vi "G4BaseTemplate_Singleton_5x6x5_GetProperty.vi"(11 "Error In":errorcluster) -> (8 "Property":dbl, 15 "Error Out":errorcluster)   [LabVIEW 2020]
uses:
  <resource>/Framework/Providers/Open_GDS/ClassProviders/Provider_EndevoGOOP400/Templates/G4BaseTemplate_Singleton_5x6x5/G4BaseTemplate_Singleton_5x6x5.lvclass
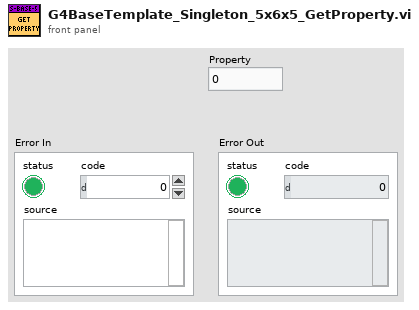
[diagram p1: front panel]
types:
  T1 = typedef "G4BaseTemplate_Singleton_5x6x5.lvclass/ObjectAttributes.ctl" = cluster{"Attribute1":dbl}
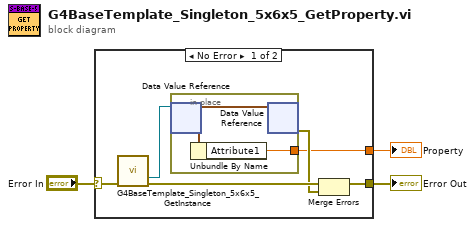
[diagram p0: block diagram]
diagram:
  n1 = case shown="No Error" "Error In" {
    selector: "Error In" -> [w9 w12]
    tunnel: [w7 w12] -> w2
    tunnel: [w5 _] -> w1
    frame No Error {
      n2 = call <resource>:"G4BaseTemplate_Singleton_5x6x5_GetInstance.vi"("error in"=w9) -> ("DVRRefOut"=w4:refnum<data-value>, "error out"=w8:errorcluster)  [unwired: 10 in, 3 out]
      n3 = in-place {
        in-place-border: [w11] -> w5
        n4 = in-place-dvr #1(w4) -> (w10:T1)  [unwired: 1 out]
        n5 = Unbundle By Name(w10) -> ("Attribute1"=w11:dbl)
        n6 = in-place-dvr #1(w10) -> (w6:errorcluster)  [unwired: 1 out]
      }
      n7 = Merge Errors(w8, w6) -> (w7:errorcluster)
    }
    frame Error {
    }
  }
  "Error Out" <- w2
  "Property" <- w1
